vi "Build Support.vi"() -> ()   [LabVIEW 2012]
uses:
  <vilib>/zip/NI_Unzip.lvlib
panel:
  out "error out":errorcluster
  in  "Variant":variant
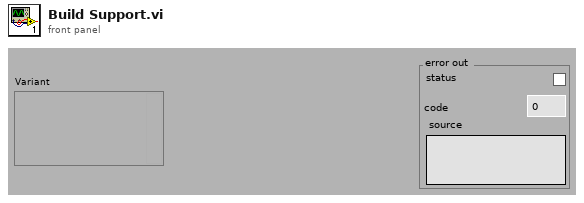
[diagram p1: front panel]
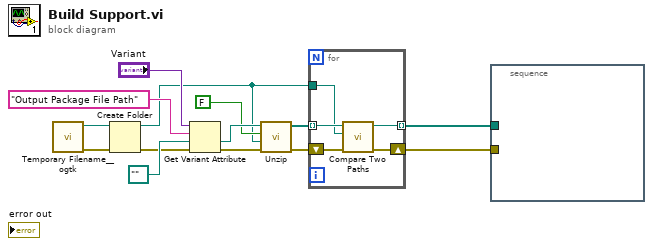
[diagram p0: block diagram]
diagram:
  n1 = call <userlib>:"Temporary Filename__ogtk.vi"() -> ("error out"=w9:errorcluster, "file in tmp dir"=w8:path)  [unwired: 3 in, 3 out]
  n2 = Create Folder(path (use dialog)=w8, error in=w9) -> (created path=w5:path, error out=w3:errorcluster)  [unwired: 2 out]
  n3 = Get Variant Attribute(Variant="Variant", name="Output Package File Path", default value (empty Variant)=path "" ("Zip file"), error in=w3) -> (value=w11:path, error out=w10:errorcluster)  [unwired: 2 out]
  n4 = call <vilib>:"Unzip.vi"("error in (no error)"=w10, "Target directory (same as Zip file if empty)"=w5, "Preview only?"=FALSE, "Zip file"=w11) -> ("error out"=w4:errorcluster, "Unzipped files"=w6:path[])  [unwired: 6 out]
  n5 = for {
    tunnel: w6 -> [w19] mode=indexing
    tunnel: w5 -> [w18]
    shift-right: [w16] -> w2
    shift-left: w4 -> [w17]
    tunnel: [w15] -> w1 mode=indexing
    n6 = call <vilib>:"Compare Two Paths.vi"("error in (no error)"=w17, "Path 2"=w18, "Path 1"=w19) -> ("error out"=w16:errorcluster, "Relative Path from 1 to 2"=w15:path)  [unwired: 7 out]
  }
  n7 = stacked-sequence {
    tunnel: w2 -> [_]
    tunnel: w1 -> [_]
    frame #0 {
    }
  }
